vi "Integer LabVIEW Code Generation.vi"() -> ()   [LabVIEW 2023]
doc: "Demonstrates how to use the DFD FXP Code Generator VI to generate integer LabVIEW code from a fixed-point filter.\n\nComplete the following steps to use this VI.\n1) Select a filter structure from <B>Target Structure</B>.\n2) Specify a <B>Destination Folder</B> for code generation.\n3) Specify a <B>Filter Name</B> for code generation.\n4) Specify <B># Channels</B> that you want the filter to process.\n5) Specify <B>Open Project?</B> to decide whether to open the generated LabVIEW project or not after code generation.\n6) Run the VI.\n7) Open the generated LabVIEW project (.lvproj) file to view the generated fixed-point filter block.\n\n<B>Note:</B> Refer to the LabVIEW Help for information about restrictions on generating code from fixed-point filters."
uses:
  <vilib>/addons/Digital Filter Design/FXPModel.llb/DFD FXP Quantize Coef (Easy).vi
  <vilib>/addons/Digital Filter Design/CodeGen.llb/DFD FXP Integer LabVIEW Code Generator.vi
  <vilib>/addons/Digital Filter Design/NI_DigFilterLicensed.lvlib
panel:
  in  "Open Project?":bool=TRUE
  in  "# Channels":i32=1
  in  "Filter Name":string
  in  "Destination Folder":path
  out "lvproj Path":path
  out "Error Message":string
  in  "Target Structure":u16(ring)=1 items=["FIR Direct Form"=1, "FIR Direct Form Transposed"=2, "FIR Symmetric"=3, "FIR Antisymmetric"=4, "IIR Direct Form I"=5, "IIR Direct Form I Transposed"=6, "IIR Direct Form II"=7, "IIR Direct Form II Transposed"=8, "IIR Cascaded Second-Order Sections Form I"=9, "IIR Cascaded Second-Order Sections Form I Transposed"=10, "IIR Cascaded Second-Order Sections Form II"=11, "IIR Cascaded Second-Order Sections Form II Transposed"=12, "Lattice Allpass (basic sections)"=13, "Lattice Allpass (one multiplier sections)"=14, "Lattice Allpass (normalized sections)"=15, "Lattice AR (basic sections)"=16, "Lattice AR (one multiplier sections)"=17, "Lattice AR (normalized sections)"=18, "Lattice MA (minimum phase)"=19, "Lattice MA (maximum phase)"=20, "Lattice ARMA (basic sections)"=21, "Lattice ARMA (one multiplier sections)"=22, "Lattice ARMA (normalized sections)"=23]
  # "Select Help>>Show Context Help and move the cursor over the VI icon for more information."
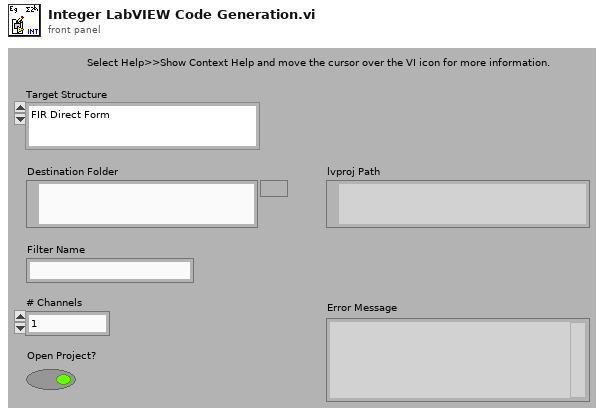
[diagram p1: front panel]
types:
  T1 = enum16{"Butterworth", "Chebyshev", "Inverse Chebyshev", "Elliptic", "Kaiser Window", "Dolph-Chebyshev Window", "Equi-Ripple FIR"}
  T2 = typedef "NI_DigFilterLicensed.lvlib/DFD Filter Obj.ctl" = cluster{"mSRate_Fs":dbl, "mSRate_Version":string, "mSRate_Comments":string, "mSRate_OrgCoef":T3, "mSRate_CurCoef":T3, "mSRate_Quantized?":bool, "mSRate_QCoef":T3, "mSRate_QSettings":T5[], "mSRate_Order":i32, "mSRate_Scaling":cluster{"mSRate_ScaleByPowerOf2?":bool, "mSRate_ScaleType":T7}}
  T3 = typedef "NI_DigFilterLicensed.lvlib/DFD Filter Coef.ctl" = cluster{"type":T4, "gain":dbl, "coef a (k)":dbl[], "coef b (v)":dbl[]}
  T4 = typedef "NI_DigFilterLicensed.lvlib/DFD Filter Structure Type Selector.ctl" = enum16{"Undefined", "FIR Direct Form", "FIR Direct Form Transposed", "FIR Symmetric", "FIR Antisymmetric", "IIR Direct Form I", "IIR Direct Form I Transposed", "IIR Direct Form II", "IIR Direct Form II Transposed", "IIR Cascaded Second Order Sections Form I", "IIR Cascaded Second Order Sections Form I Transposed", "IIR Cascaded Second Order Sections Form II", "IIR Cascaded Second Order Sections Form II Transposed", "Lattice Allpass (basic sections)", "Lattice Allpass (one multiplier sections)", "Lattice Allpass (normalized sections)", "Lattice AR (basic sections)", "Lattice AR (one multiplier sections)", "Lattice AR (normalized sections)", "Lattice MA (minimum phase)", "Lattice MA (maximum phase)", "Lattice ARMA (basic sections)", "Lattice ARMA (one multiplier sections)", "Lattice ARMA (normalized sections)"}
  T5 = typedef "NI_DigFilterLicensed.lvlib/dfd_Internal Quantization Settings.ctl" = cluster{"source":T6, "wl":i16, "iwl":i16, "overflow mode":enum16{"Saturation", "Wrap"}, "rounding mode":enum16{"Nearest", "Truncation"}, "signed?":bool}
  T6 = typedef "NI_DigFilterLicensed.lvlib/dfd_Internal Quantization Srcs.ctl" = u16
  T7 = typedef "NI_DigFilterLicensed.lvlib/DFD Coef Norm Type.ctl" = enum16{"No Norm", "Time Domain 1-Norm", "Time Domain 2-Norm", "Time Domain Inf-Norm"}
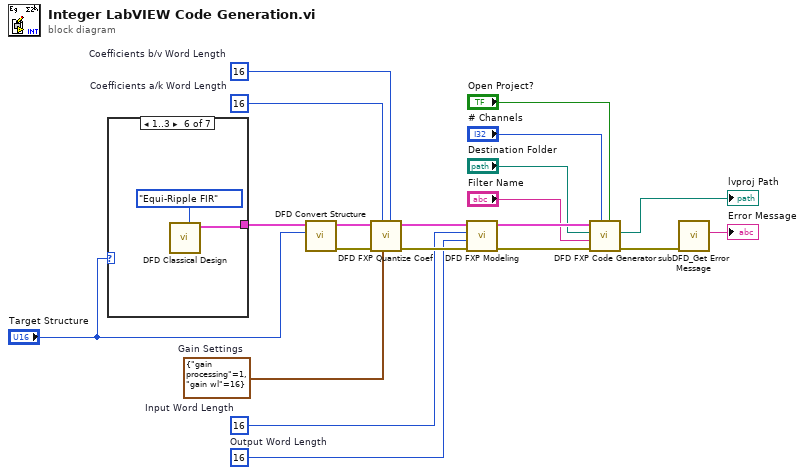
[diagram p0: block diagram]
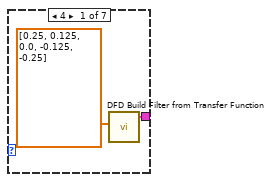
[diagram p2: hidden frame]
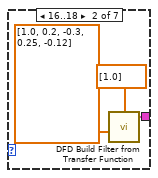
[diagram p3: hidden frame]
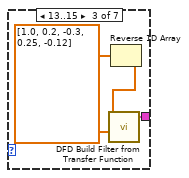
[diagram p4: hidden frame]
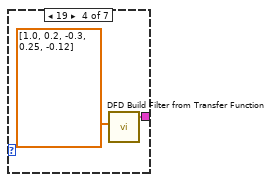
[diagram p5: hidden frame]
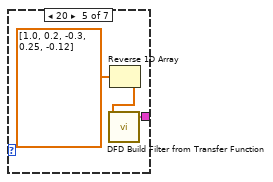
[diagram p6: hidden frame]
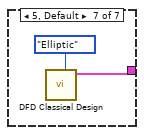
[diagram p7: hidden frame]
diagram:
  w1 = i16 16  # Output Word Length
  w2 = i16 16  # Input Word Length
  w13 = cluster{"gain processing":u16, "gain wl":i16} {"gain processing"=1, "gain wl"=16}  # Gain Settings
  w14 = i16 16  # Coefficients b/v Word Length
  w15 = i16 16  # Coefficients a/k Word Length
  n1 = case shown="1..3" "Target Structure" {
    tunnel: [w22 w25 w28 w30 w33 w35 w37] -> w20
    frame 4 {
      n2 = call <vilib>:"DFD Build Filter from Transfer Function.vi"("numerator"=dbl[] [0.25, 0.125, 0.0, -0.125, -0.25]) -> ("filter out"=w22:T2)  [unwired: 3 in, 7 out]
    }
    frame 16..18 {
      n3 = call <vilib>:"DFD Build Filter from Transfer Function.vi"("denominator"=dbl[] [1.0, 0.2, -0.3, 0.25, -0.12] ("numerator"), "numerator"=dbl[] [1.0]) -> ("filter out"=w25:T2)  [unwired: 2 in, 7 out]
    }
    frame 13..15 {
      w27 = dbl[] [1.0, 0.2, -0.3, 0.25, -0.12] ("numerator")
      n4 = Reverse 1D Array(array=w27) -> (reversed array=w26:dbl[])
      n5 = call <vilib>:"DFD Build Filter from Transfer Function.vi"("denominator"=w27, "numerator"=w26) -> ("filter out"=w28:T2)  [unwired: 2 in, 7 out]
    }
    frame 19 {
      n6 = call <vilib>:"DFD Build Filter from Transfer Function.vi"("numerator"=dbl[] [1.0, 0.2, -0.3, 0.25, -0.12]) -> ("filter out"=w30:T2)  [unwired: 3 in, 7 out]
    }
    frame 20 {
      n7 = Reverse 1D Array(array=dbl[] [1.0, 0.2, -0.3, 0.25, -0.12] ("numerator")) -> (reversed array=w31:dbl[])
      n8 = call <vilib>:"DFD Build Filter from Transfer Function.vi"("numerator"=w31) -> ("filter out"=w33:T2)  [unwired: 3 in, 7 out]
    }
    frame 1..3 {
      n9 = call <vilib>:"DFD Classical Design.vi"("design method"=T1."Equi-Ripple FIR") -> ("filter out"=w35:T2)  [unwired: 5 in, 5 out]
    }
    frame 5, Default {
      n10 = call <vilib>:"DFD Classical Design.vi"("design method"=T1."Elliptic") -> ("filter out"=w37:T2)  [unwired: 5 in, 5 out]
    }
  }
  n11 = call <vilib>:"DFD Convert Structure.vi"("target structure"="Target Structure", "filter in"=w20) -> ("error out"=w16:errorcluster, "filter out"=w17:T2)  [unwired: 1 in, 7 out]
  n12 = call-poly <vilib>:"DFD FXP Quantize Coef.vi"("coefficients b/v word length"=w14, "gain settings"=w13, "coefficients a/k word length"=w15, "error in (no error)"=w16, "filter in"=w17) -> ("error out"=w11:errorcluster, "filter out"=w12:T2)  [unwired: 5 out]
  n13 = call <vilib>:"DFD FXP Modeling.vi"("error in (no error)"=w11, "output word length"=w1, "input word length"=w2, "filter in"=w12) -> ("error out"=w9:errorcluster, "filter out"=w10:T2)  [unwired: 3 in, 3 out]
  n14 = call-poly <vilib>:"DFD FXP Code Generator.vi"("open project? (F)"="Open Project?", "# channels"="# Channels", "error in (no error)"=w9, "filter name"="Filter Name", "destination folder"="Destination Folder", "filter in"=w10) -> ("error out"=w8:errorcluster, "lvproj path"=→"lvproj Path":path)  [unwired: 1 in, 3 out]
  n15 = call <vilib>:"subDFD_Get Error Message.vi"("error in (no error)"=w8) -> ("Error Message"=→"Error Message":string)  [unwired: 10 out]
